vi "BenchmarkParams.vi"() -> (0 "error out":errorcluster, 3 "Numeric":dbl)   [LabVIEW 2012]
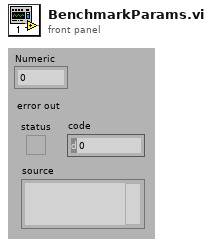
[diagram p1: front panel]
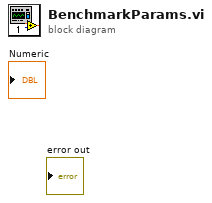
[diagram p0: block diagram]
diagram:
